vi "Parse Injection Data.vi"(10 "Injection.Results":T12 {"Measurements"."Shots"."Results"."Off-Stage Min Volt" format="%#.6g"; "Measurements"."Shots"."Results"."Off-Stage Avg Volt" format="%#.6g"; "Measurements"."Shots"."Results"."Off-Stage Max Volt" format="%#.6g"; "Measurements"."Shots"."Results"."Total Stage Time (us)" format="%#.6g"; "Measurements"."Shots"."Results"."Off-Stage Avg Current" format="%#.6g"; "Measurements"."Shots"."Results"."Total Voltage Pulses" format="%#.6g"; "Measurements"."Shots"."Results"."Off-Stage Min Current" format="%#.6g"; "Measurements"."Shots"."Results"."Off-Stage Max Current" format="%#.6g"}, 11 "Parameters":T1) -> (2 "Injection.Results":T12 {"Measurements"."Shots"."Results"."Off-Stage Min Volt" format="%#.6g"; "Measurements"."Shots"."Results"."Off-Stage Avg Volt" format="%#.6g"; "Measurements"."Shots"."Results"."Off-Stage Max Volt" format="%#.6g"; "Measurements"."Shots"."Results"."Total Stage Time (us)" format="%#.6g"; "Measurements"."Shots"."Results"."Off-Stage Avg Current" format="%#.6g"; "Measurements"."Shots"."Results"."Total Voltage Pulses" format="%#.6g"; "Measurements"."Shots"."Results"."Off-Stage Min Current" format="%#.6g"; "Measurements"."Shots"."Results"."Off-Stage Max Current" format="%#.6g"}, 3 "Parameters":T1)   [LabVIEW 2015, in "Fuel Injector Analysis Addon Engine.lvlib"]
uses:
  Fuel Injector Analysis Addon Engine.lvlib
  Types/Injector Event Data Cluster.ctl
  RT Analysis/Controls/Shot Information Control.ctl
  Types/Stage.Measurements.ctl
  Types/Async Parameters.ctl
  Shared/Types/Shot.Parameters.ctl
  Shared/Types/Stage.Parameters.ctl
  Shared/Types/Stage.PullIn.Types.ctl
  Shared/Types/Stage.Transition.Types.ctl
  Shared/Types/Analysis.Channels.Select.ctl
  Shared/Types/Injector info.ctl
  Types/Injector.State.ctl
  <vilib>/NI/NIVS Inline Async API/_Data Access Engine/Data Access Engine/Types/Write.DVR.ctl
  <vilib>/NI/NIVS Inline Async API/_Data Access Engine/Access Type Classes/Write/Write.lvclass
  <vilib>/NI/NIVS Inline Async API/_Data Access Engine/Data Access Engine/Types/Read.DVR.ctl
  <vilib>/NI/NIVS Inline Async API/_Data Access Engine/Access Type Classes/Read/Read.lvclass
  <vilib>/NI Veristand/Custom Device API/Waveform Data Reference.ctl
  <vilib>/NI VeriStand/Custom Device Waveform API/Single Waveform Write (DBL)/Single Waveform Write (DBL).lvclass
  Shared/Fuel Injector Analysis Addon Shared.lvlib
  <vilib>/NI Veristand/Custom Device API/Custom Device API.lvlib
  <vilib>/NI/NIVS Inline Async API/_Data Access Engine/Data Access Engine/Data Access Engine.lvclass
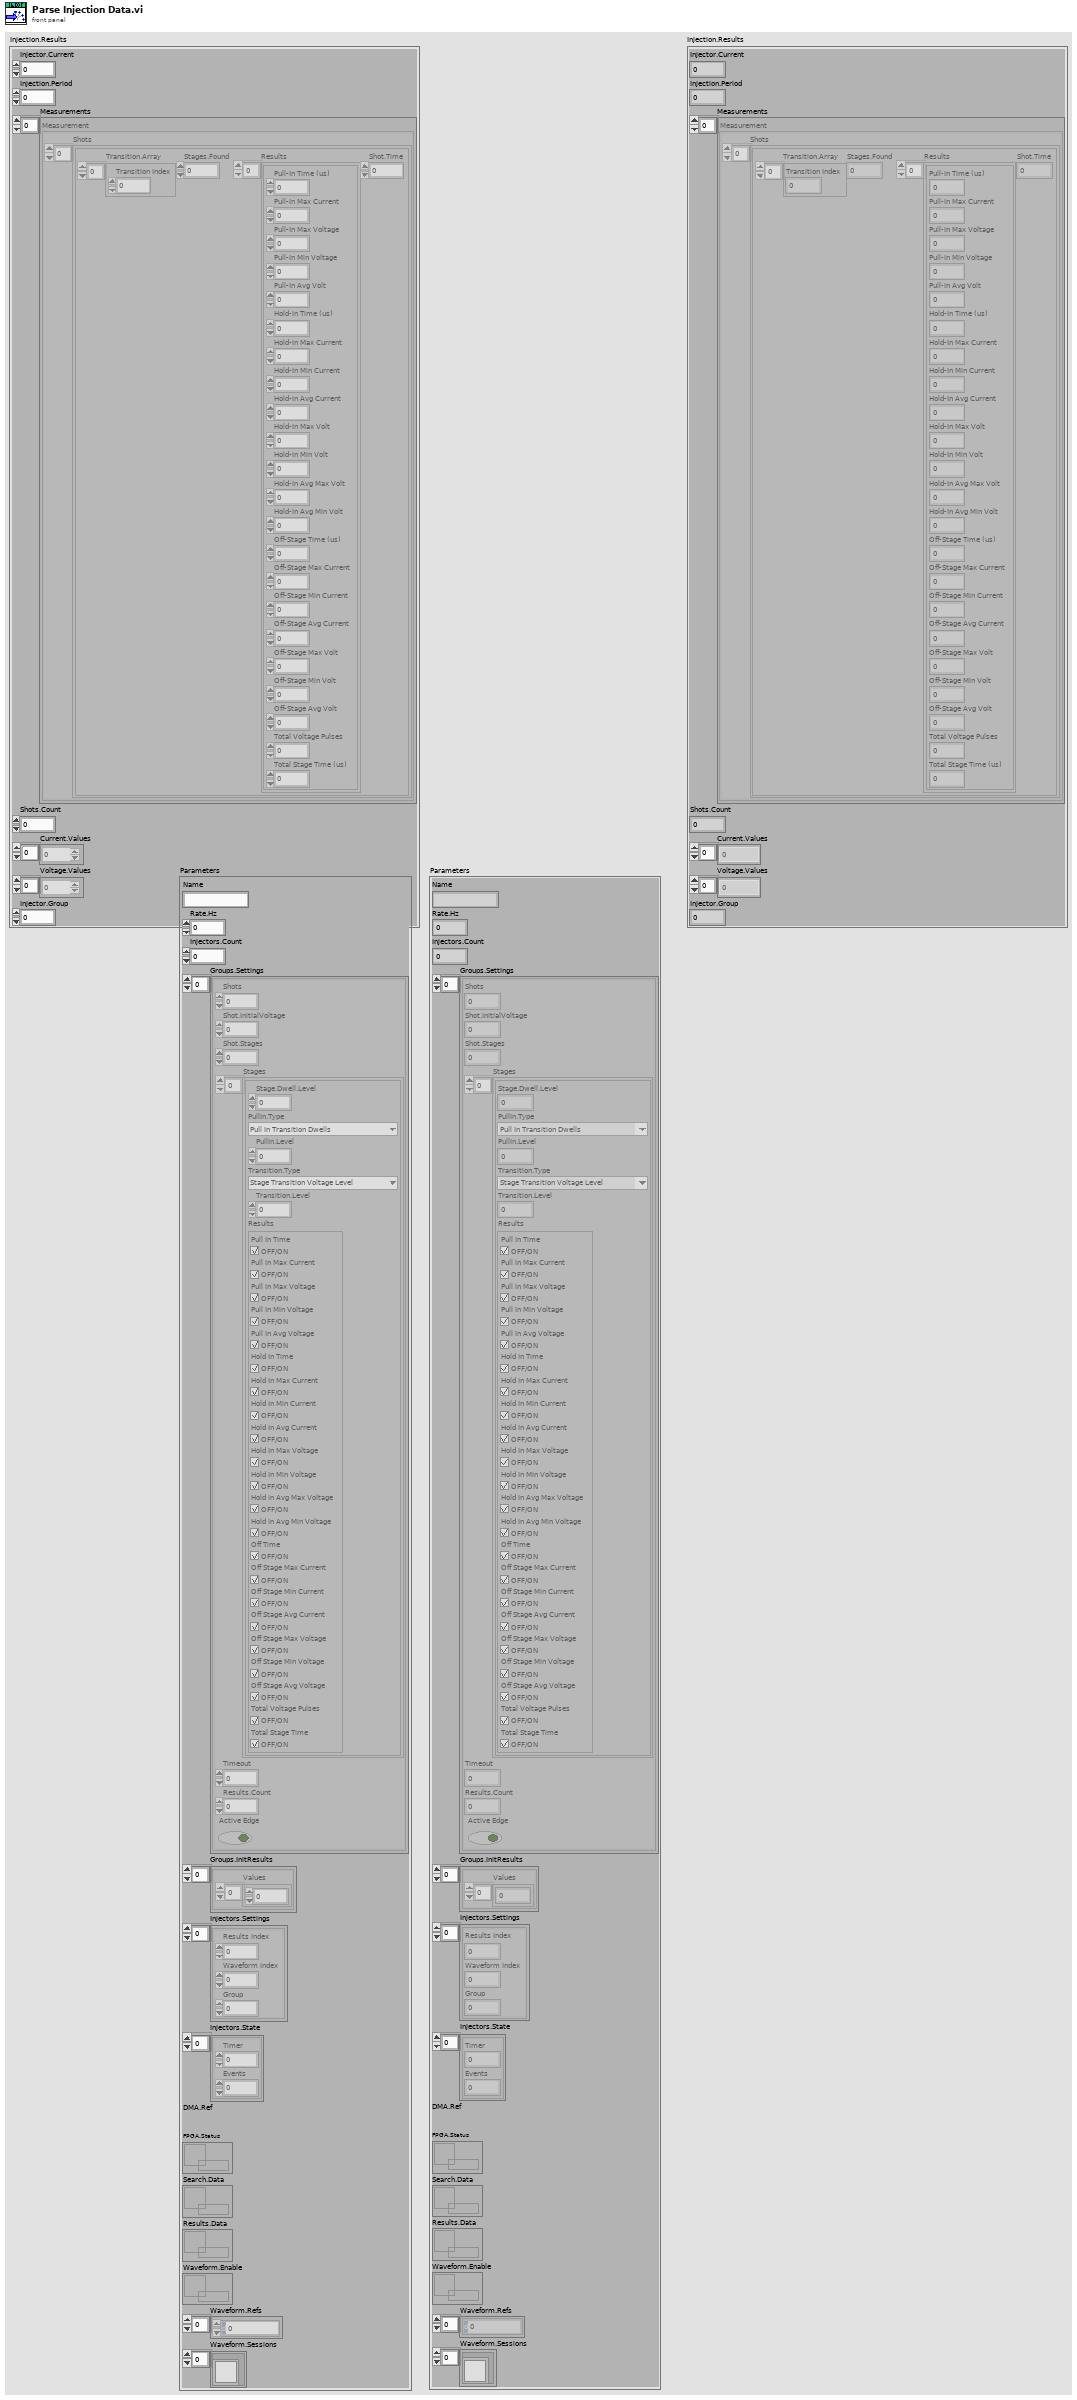
[diagram p1: front panel]
types:
  T1 = typedef "Fuel Injector Analysis Addon Engine.lvlib/Async Parameters.ctl" = cluster{"Name":string, "Rate.Hz":u32, "Injectors.Count":u8, "Groups.Settings":T2[], "Groups.InitResults":cluster{"Values":dbl[]}[], "Injectors.Settings":T7[], "Injectors.State":T8[], "DMA.Ref":refnum<k20>, "FPGA.Status":T9, "Search.Data":T10, "Results.Data":T9, "Waveform.Enable":T10, "Waveform.Refs":T11[], "Waveform.Sessions":refnum<class "Single Waveform Write (DBL).lvclass">[]}
  T2 = typedef "Fuel Injector Analysis Addon Shared.lvlib/Shot.Parameters.ctl" = cluster{"Shots":u32, "Shot.InitialVoltage":dbl, "Shot.Stages":u32, "Stages":T3[], "Timeout":dbl, "Results.Count":i32, "Active Edge":bool}
  T3 = typedef "Fuel Injector Analysis Addon Shared.lvlib/Stage.Parameters.ctl" = cluster{"Stage.Dwell.Level":dbl, "PullIn.Type":T4, "PullIn.Level":dbl, "Transition.Type":T5, "Transition.Level":dbl, "Results":T6}
  T4 = typedef "Fuel Injector Analysis Addon Shared.lvlib/Stage.PullIn.Types.ctl" = enum8{"Pull In Transition Dwells", "Pull In Transition Current Drop"}
  T5 = typedef "Fuel Injector Analysis Addon Shared.lvlib/Stage.Transition.Types.ctl" = enum8{"Stage Transition Dwell Time", "Stage Transition Voltage Level", "Stage Transition Current Drop", "Stage Transition Active Time"}
  T6 = typedef "Fuel Injector Analysis Addon Shared.lvlib/Analysis.Channels.Select.ctl" = cluster{"Pull In Time":bool, "Pull In Max Current":bool, "Pull In Max Voltage":bool, "Pull In Min Voltage":bool, "Pull In Avg Voltage":bool, "Hold In Time":bool, "Hold In Max Current":bool, "Hold In Min Current":bool, "Hold In Avg Current":bool, "Hold In Max Voltage":bool, "Hold In Min Voltage":bool, "Hold In Avg Max Voltage":bool, "Hold In Avg Min Voltage":bool, "Off Time":bool, "Off Stage Max Current":bool, "Off Stage Min Current":bool, "Off Stage Avg Current":bool, "Off Stage Max Voltage":bool, "Off Stage Min Voltage":bool, "Off Stage Avg Voltage":bool, "Total Voltage Pulses":bool, "Total Stage Time":bool}
  T7 = typedef "Fuel Injector Analysis Addon Shared.lvlib/Injector info.ctl" = cluster{"Results Index":i32, "Waveform Index":i32, "Group":u16}
  T8 = typedef "Fuel Injector Analysis Addon Engine.lvlib/Injector.State.ctl" = cluster{"Timer":u32, "Events":u64}
  T9 = typedef "Data Access Engine.lvlib/Data Access Engine.lvclass/Write.DVR.ctl" = refnum<data-value>
  T10 = typedef "Data Access Engine.lvlib/Data Access Engine.lvclass/Read.DVR.ctl" = refnum<data-value>
  T11 = typedef "Custom Device API.lvlib/Waveform Data Reference.ctl" = i32
  T12 = typedef "Fuel Injector Analysis Addon Engine.lvlib/Injector Event Data Cluster.ctl" = cluster{"Injector.Current":i16, "Injection.Period":dbl, "Measurements":cluster{"Shots":T13[]}[], "Shots.Count":i32, "Current.Values":dbl[], "Voltage.Values":dbl[], "Injector.Group":i16}
  T13 = typedef "Fuel Injector Analysis Addon Engine.lvlib/Shot Information Control.ctl" = cluster{"Transition.Array":i32[], "Stages.Found":u16, "Results":T14[], "Shot.Time":dbl}
  T14 = typedef "Fuel Injector Analysis Addon Engine.lvlib/Stage.Measurements.ctl" = cluster{"Pull-In Time (us)":dbl, "Pull-In Max Current":dbl, "Pull-In Max Voltage":dbl, "Pull-In Min Voltage":dbl, "Pull-In Avg Volt":dbl, "Hold-In Time (us)":dbl, "Hold-In Max Current":dbl, "Hold-In Min Current":dbl, "Hold-In Avg Current":dbl, "Hold-In Max Volt":dbl, "Hold-In Min Volt":dbl, "Hold-In Avg Max Volt":dbl, "Hold-In Avg Min Volt":dbl, "Off-Stage Time (us)":dbl, "Off-Stage Max Current":dbl, "Off-Stage Min Current":dbl, "Off-Stage Avg Current":dbl, "Off-Stage Max Volt":dbl, "Off-Stage Min Volt":dbl, "Off-Stage Avg Volt":dbl, "Total Voltage Pulses":dbl, "Total Stage Time (us)":dbl}
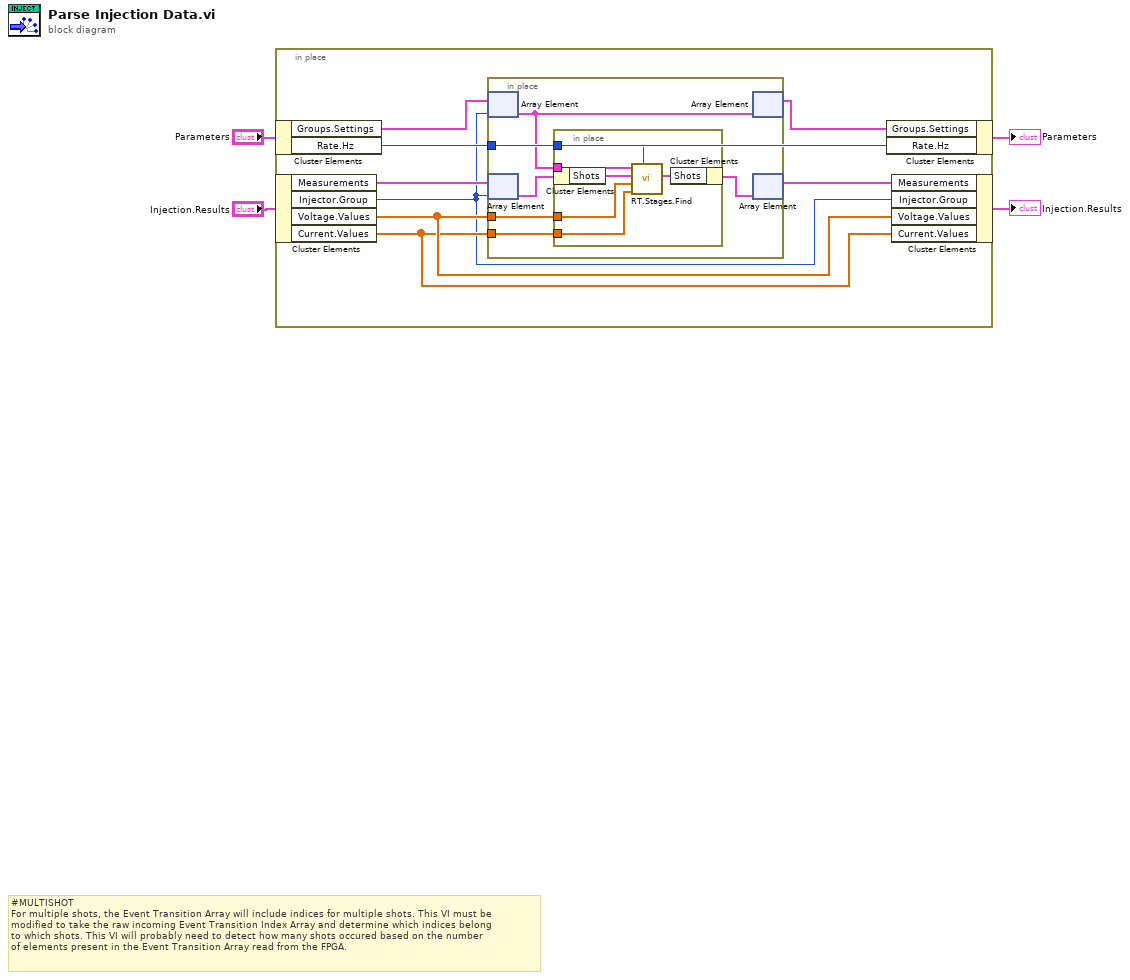
[diagram p0: block diagram]
diagram:
  # "#MULTISHOT\nFor multiple shots, the Event Transition Array will include indices for multiple shots. This VI must be \nmodified to take the raw incoming Event Transition Index Array and determine which indices belong\nto which shots. This VI will probably need to detect how many shots occured based on the number\nof elements present in the Event Transition Array read from the FPGA."
  n1 = in-place {
    n2 = in-place-cluster #1("Parameters") -> ("Groups.Settings"=w8:T2[], "Rate.Hz"=w10:u32)
    n3 = in-place-cluster #2("Injection.Results") -> ("Measurements"=w9:cluster{"Shots":T13[]}[], "Injector.Group"=w5:i16, "Voltage.Values"=w12:dbl[], "Current.Values"=w11:dbl[])
    n4 = in-place {
      in-place-border: w12 -> [w18]
      in-place-border: w11 -> [w17]
      in-place-border: w10 -> [w16]
      n5 = in-place-array #3(w8, w5) -> (w13:T2)
      n6 = in-place-array #4(w9, w5) -> (w15:cluster{"Shots":T13[]})
      n7 = in-place {
        in-place-border: w18 -> [w24]
        in-place-border: w17 -> [w23]
        in-place-border: w16 -> [w22]
        in-place-border: w13 -> [w20]
        n8 = in-place-cluster #5(w15) -> ("Shots"=w21:T13[])
        n9 = call "RT.Stages.Find.vi"("Rate.Hz"=w22, "Current Data"=w23, "Voltage Data"=w24, "Shots"=w21, "Parameters"=w20) -> ("Shots"=w19:T13[])  [unwired: 6 in]
        n10 = in-place-cluster #5("Shots"=w19) -> (w14:cluster{"Shots":T13[]})
      }
      n11 = in-place-array #3(w13) -> (w6:T2[])  [unwired: 1 out]
      n12 = in-place-array #4(w14) -> (w7:cluster{"Shots":T13[]}[])  [unwired: 1 out]
    }
    n13 = in-place-cluster #1("Groups.Settings"=w6, "Rate.Hz"=w10) -> (→"Parameters":T1)
    n14 = in-place-cluster #2("Measurements"=w7, "Injector.Group"=w5, "Voltage.Values"=w12, "Current.Values"=w11) -> (→"Injection.Results":T12)
  }
